vi "写入data.vi"(8 "error in (no error)":errorcluster caption="错误输入（无错误）", 10 "data":T1, 11 "LS-H600-TCP Client输入":refnum<class "LS-H600-TCP Client.lvclass">) -> (0 "error out":errorcluster caption="错误输出", 3 "LS-H600-TCP Client输出":refnum<class "LS-H600-TCP Client.lvclass">)   [LabVIEW 2022 SP3, in "LS-H600-TCP Client.lvlib" / "LS-H600-TCP Client.lvclass"]
uses:
  LS-H600-TCP Client.lvclass
  LS-H600-TCP Client.lvclass/LS-H600-TCP Client.ctl
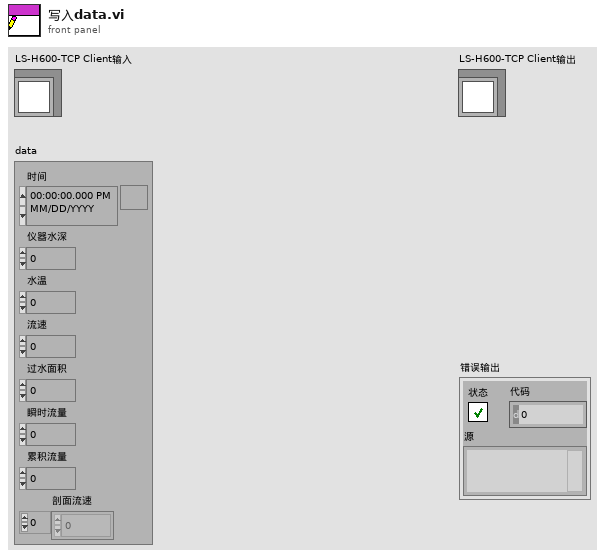
[diagram p1: front panel]
types:
  T1 = cluster{"时间":timestamp, "仪器水深":dbl, "水温":dbl, "流速":dbl, "过水面积":dbl, "瞬时流量":dbl, "累积流量":dbl, "剖面流速":dbl[]}
  T2 = cluster{"数据输出":string, "data":cluster{"时间":timestamp, "仪器水深":dbl, "水温":dbl, "流速":dbl, "过水面积":dbl, "瞬时流量":dbl, "累积流量":dbl, "剖面流速":dbl[]}, "连接错误":errorcluster}
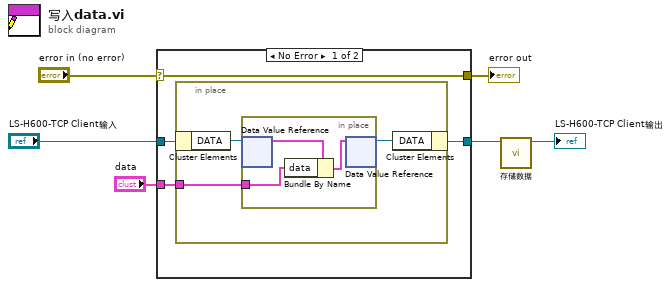
[diagram p0: block diagram]
diagram:
  n1 = case shown="No Error" "error in (no error)" {
    selector: "error in (no error)" -> [w10 w17]
    tunnel: [w10 w17] -> w5
    tunnel: [w8 w18] -> w2
    tunnel: "LS-H600-TCP Client输入" -> [w9 w18]
    tunnel: "data" -> [w7 _]
    frame No Error {
      n2 = in-place {
        in-place-border: w7 -> [w12]
        n3 = in-place-cluster #1(w9) -> ("DATA"=w13:refnum<data-value>)
        n4 = in-place {
          in-place-border: w12 -> [w15]
          n5 = in-place-dvr #2(w13) -> (w16:T2)  [unwired: 1 out]
          n6 = Bundle By Name(cluster=w16, "data"=w15) -> (w14:T2)
          n7 = in-place-dvr #2(w14) -> (w11:refnum<data-value>)  [unwired: 1 out]
        }
        n8 = in-place-cluster #1("DATA"=w11) -> (w8:refnum<class "LS-H600-TCP Client.lvclass">)
      }
    }
    frame Error {
    }
  }
  "error out" <- w5
  n9 = call "存储数据.vi"("LS-H600-TCP Client 输入"=w2) -> ("LS-H600-TCP Client 输出"=→"LS-H600-TCP Client输出":refnum<class "LS-H600-TCP Client.lvclass">)  [unwired: 9 in, 1 out]
